vi "CMD_POTDOT.vi"(6 "Gantry in":refnum<class "Gantry.lvclass">, 8 "error in (no error)":errorcluster, 10 "Arguments":string[](array[string]), 11 "gScript Interpreter in":refnum<class "gScript Interpreter.lvclass">) -> (0 "error out":errorcluster, 3 "gScript Interpreter out":refnum<class "gScript Interpreter.lvclass">, 4 "Gantry out":refnum<class "Gantry.lvclass">)   [LabVIEW 2023, in "gScript Interpreter.lvclass"]
uses:
  gScript Interpreter.lvclass
  Shared Components/Gantry Class/Gantry.lvclass
  Shared Components/FlexWorktable/FlexWorktable.lvclass
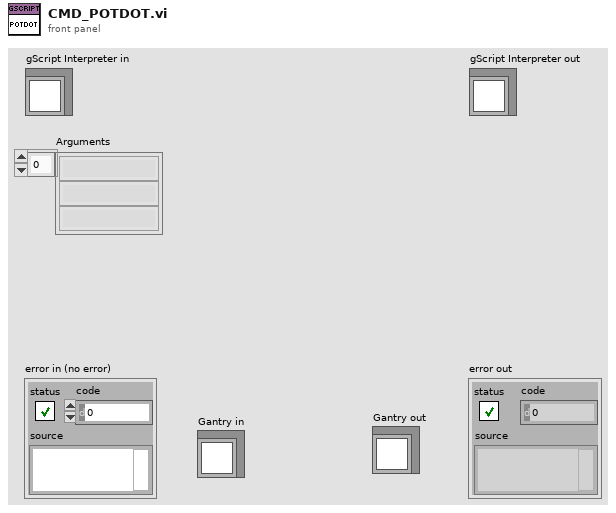
[diagram p1: front panel]
types:
  T1 = typedef "Memory Cell.ctl" = cluster{"type":T2, "x":dbl, "y":dbl, "z":dbl, "w":dbl}
  T2 = typedef "Memory Cell Type Enum.ctl" = enum16{"integer", "float", "vector", "rotation"}
  T3 = cluster{"Syringe Holder":string, "Mixing Time":timestamp, "Tip Offset":refnum<class "Vec3d.lvclass">}
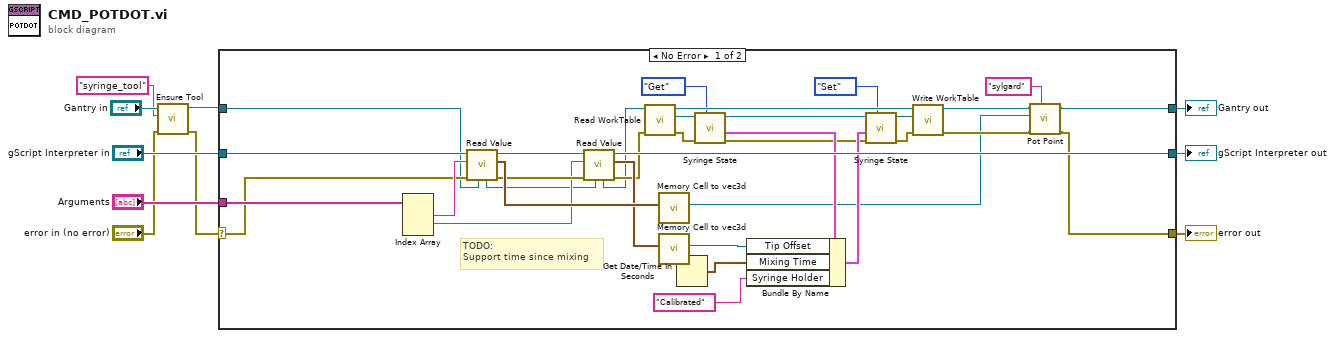
[diagram p0: block diagram]
diagram:
  n1 = call "Ensure Tool.vi"("error in (no error)"="error in (no error)", "Tool Name"="syringe_tool", "Gantry in"="Gantry in") -> ("error out"=w2:errorcluster, "Gantry out"=w4:refnum<class "Gantry.lvclass">)  [unwired: 7 in]
  n2 = case shown="No Error" w2 {
    selector: w2 -> [w14 w47]
    tunnel: [w40 w47] -> w10
    tunnel: [w42 w46] -> w8
    tunnel: "gScript Interpreter in" -> [w43 w46]
    tunnel: "Arguments" -> [w44 _]
    tunnel: w4 -> [w13 w45]
    tunnel: [w41 w45] -> w5
    frame No Error {
      # "TODO:\nSupport time since mixing"
      n3 = Index Array(array=w44) -> (element #1=w39:string, element #2=w30:string)  [unwired: 3 in, 1 out]
      n4 = call-dynamic "Read Value.vi"("Gantry in"=w13, "error in (no error)"=w14, "String in"=w39, "gScript Interpreter in"=w43) -> ("error out"=w31:errorcluster, "Memory Cell"=w38:T1, "gScript Interpreter out"=w32:refnum<class "gScript Interpreter.lvclass">, "Gantry out"=w12:refnum<class "Gantry.lvclass">)  [unwired: 4 in]
      n5 = call-dynamic "Read Value.vi"("Gantry in"=w12, "error in (no error)"=w31, "String in"=w30, "gScript Interpreter in"=w32) -> ("error out"=w21:errorcluster, "Memory Cell"=w36:T1, "gScript Interpreter out"=w42:refnum<class "gScript Interpreter.lvclass">, "Gantry out"=w11:refnum<class "Gantry.lvclass">)  [unwired: 4 in]
      n6 = call-dynamic "Read WorkTable.vi"("error in"=w21, "Gantry Class in"=w11) -> ("error out"=w20:errorcluster, "Worktable"=w29:refnum<class "FlexWorktable.lvclass">, "Gantry Class out"=w37:refnum<class "Gantry.lvclass">)  [unwired: 7 in]
      n7 = call "Memory Cell to vec3d.vi"("Memory Cell"=w38) -> ("Vec3d out"=w15:refnum<class "Vec3d.lvclass">)  [unwired: 10 in]
      n8 = call "Memory Cell to vec3d.vi"("Memory Cell"=w36) -> ("Vec3d out"=w35:refnum<class "Vec3d.lvclass">)  [unwired: 10 in]
      n9 = Get Date/Time In Seconds() -> (seconds since 1Jan1904=w34:timestamp)
      n10 = call-dynamic "Syringe State.vi"("Get/Set"=enum16{"Get", "Set"}."Get", "error in (no error)"=w20, "FlexWorktable in"=w29) -> ("error out"=w19:errorcluster, "Syringe out"=w27:T3, "FlexWorktable out"=w26:refnum<class "FlexWorktable.lvclass">)  [unwired: 6 in]
      n11 = Bundle By Name(cluster=w27, "Tip Offset"=w35, "Mixing Time"=w34, "Syringe Holder"="Calibrated") -> (w25:T3)
      n12 = call-dynamic "Syringe State.vi"("Get/Set"=enum16{"Get", "Set"}."Set", "error in (no error)"=w19, "Syringe in"=w25, "FlexWorktable in"=w26) -> ("error out"=w23:errorcluster, "FlexWorktable out"=w24:refnum<class "FlexWorktable.lvclass">)  [unwired: 5 in, 1 out]
      n13 = call-dynamic "Write WorkTable.vi"("error in (no error)"=w23, "FlexWorktable"=w24, "Gantry Class in"=w37) -> ("error out"=w18:errorcluster, "Gantry Class out"=w33:refnum<class "Gantry.lvclass">)  [unwired: 7 in]
      n14 = call "Pot Point.vi"("Encapsulant"="sylgard", "error in (no error)"=w18, "Point"=w15, "Gantry in"=w33) -> ("error out"=w40:errorcluster, "Gantry out"=w41:refnum<class "Gantry.lvclass">)  [unwired: 6 in]
    }
    frame Error {
    }
  }
  "error out" <- w10
  "gScript Interpreter out" <- w8
  "Gantry out" <- w5
